vi "Test.vi"() -> ()   [LabVIEW 2013, in "Data Logger.lvlib"]
uses:
  Data Logger.lvlib
  Data Logger.lvclass
  Data Logger.lvclass/Data Logger.ctl
  <vilib>/ActorFramework/Message Queue/Message Queue.lvclass/Message Queue.ctl
  Data Logger Messages/Write Signal Ref Msg/Write Signal Ref Msg.lvclass/Write Signal Ref Msg.ctl
  <vilib>/ActorFramework/Message Enqueuer/Message Enqueuer.lvclass/Message Enqueuer.ctl
  Data Logger Messages/Write Time Out Ref Msg/Write Time Out Ref Msg.lvclass/Write Time Out Ref Msg.ctl
  <vilib>/ActorFramework/Message Enqueuer/Enqueue.vi
  <vilib>/ActorFramework/Message Priority Queue/Priority Enqueue.vi
  Data Logger Messages/Write Signal Ref Msg/Write Signal Ref Msg.lvclass
  Data Logger Messages/Write Time Out Ref Msg/Write Time Out Ref Msg.lvclass
  <vilib>/ActorFramework/Stop Msg/Stop Msg.lvclass
  <vilib>/ActorFramework/Actor/Actor.lvclass
  <vilib>/ActorFramework/Message Queue/Message Queue.lvclass
panel:
  in  "Logging Interval":dbl=1.0 min=1.0 step=1.0 format="%<%H:%M:%S>t"
  out "error out":errorcluster
  out "Waveform Graph":dynamicdata(graph)
  out "n2":dbl
  out "n1":dbl
  out "Combined":dbl
  out "i":i32
  in  "stop":bool
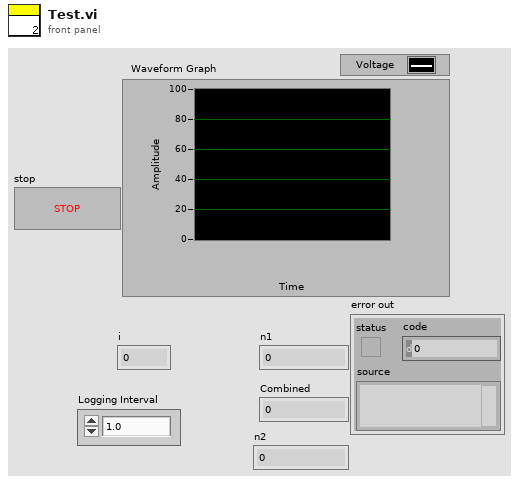
[diagram p1: front panel]
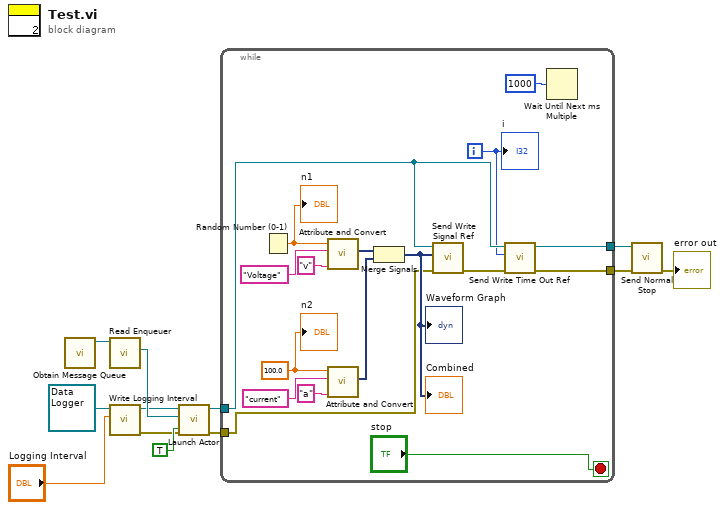
[diagram p0: block diagram]
diagram:
  n1 = call <vilib>:"Obtain Message Queue.vi"() -> ("Message Queue"=w12:refnum<class "Message Queue.lvclass">)  [unwired: 10 in, 1 out]
  n2 = call <vilib>:"Read Enqueuer.vi"("Message Queue"=w12) -> ("Message Enqueuer"=w11:refnum<class "Message Enqueuer.lvclass">)  [unwired: 10 in]
  n3 = call "Write Logging Interval.vi"("Logging Interval"="Logging Interval", "Data Logger in"=refnum<class "Data Logger.lvclass"> refnum ("Data Logger.lvlib:Data Logger.lvclass")) -> ("error out"=w2:errorcluster, "Data Logger out"=w3:refnum<class "Data Logger.lvclass">)  [unwired: 8 in]
  n4 = call <vilib>:"Launch Actor.vi"("Open Actor Core front panel? (F)"=TRUE, "error in (no error)"=w2, "Actor-to-Caller Enqueuer"=w11, "Actor"=w3) -> ("error out"=w7:errorcluster, "Caller-To-Actor Enqueuer"=w10:refnum<class "Message Enqueuer.lvclass">)  [unwired: 6 in]
  n5 = while {
    tunnel: w10 -> [w18]
    tunnel: [w17] -> w8
    tunnel: w7 -> [w14]
    tunnel: [w13] -> w6
    i -> [w16]
    stop <- "stop" stop-if-true
    w20 = 100.0 ("number (0 to 1)")
    n6 = Random Number (0-1)() -> (number: 0 to 1=w27:dbl)
    "n1" <- w27
    n7 = call "Attribute and Convert.vi"("Unit"="v", "Signal Name"="Voltage" ("Unit"), "Number in"=w27) -> ("Dynamic Signal Out"=w22:dynamicdata)  [unwired: 8 in]
    n8 = call "Attribute and Convert.vi"("Unit"="a", "Signal Name"="current", "Number in"=w20) -> ("Dynamic Signal Out"=w21:dynamicdata)  [unwired: 8 in]
    n9 = Merge Signals(w22, w21) -> (w19:dynamicdata)
    "Combined" <- w19
    "Waveform Graph" <- w19
    n10 = call "Send Write Signal Ref.vi"("error in (no error)"=w14, "Waveform Graph"=w19, "Message Enqueuer"=w18) -> ("error out"=w15:errorcluster)  [unwired: 7 in, 1 out]
    n11 = call "Send Write Time Out Ref.vi"("error in (no error)"=w15, "Numeric"=w16, "Message Enqueuer"=w18) -> ("error out"=w13:errorcluster, "Message Enqueuer out"=w17:refnum<class "Message Enqueuer.lvclass">)  [unwired: 7 in]
    n12 = Wait Until Next ms Multiple(millisecond multiple=u32 1000) -> ()  [unwired: 1 out]
    "n2" <- w20
    "i" <- w16
  }
  n13 = call <vilib>:"Send Normal Stop.vi"("error in (no error)"=w6, "Message Enqueuer"=w8) -> ("error out"=→"error out":errorcluster)  [unwired: 9 in]
